vi "Append VI List of SubVIs to Report (string).vi"(0 "report in":refnum<class "NI_report.lvclass">, 2 "image format (jpeg)":enum32{"PNG", "JPEG", "GIF"}(ring)=enum."JPEG", 5 "VI":string, 7 "alignment (default)":T2, 9 "include Express VI configuration information (F)":bool, 11 "error in (no error)":errorcluster, 12 "MS Office parameters":T1) -> (4 "report out":refnum<class "NI_report.lvclass">, 6 "VI name out":string, 8 "start out (Word)":i32, 10 "end out (Word)":i32, 15 "error out":errorcluster)   [LabVIEW 2017, in "NI_ReportGenerationCore.lvlib"]
doc: "Appends a list of subVIs of the VI you specify in <B>VI</B> to a report. The list includes subVI icons, names, and paths. Wire data to the <B>VI</B> input to determine the polymorphic instance to use or manually select the instance."
uses:
  <vilib>/Utility/NIReport.llb/NI_ReportGenerationCore.lvlib
  <vilib>/Utility/NIReport.llb/NI_report.lvclass
  <vilib>/Utility/NIReport.llb/HTML Report Image Alignment.ctl
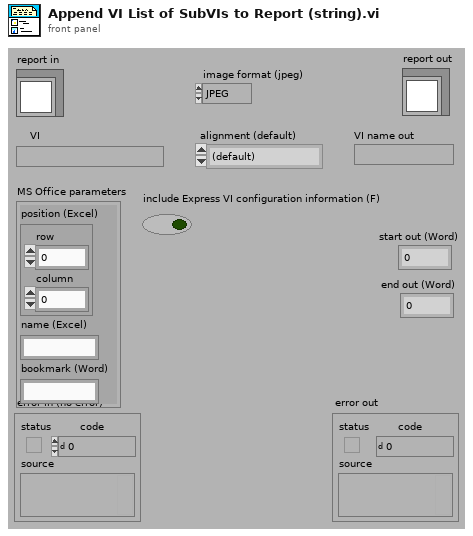
[diagram p1: front panel]
types:
  T1 = cluster{"position (Excel)":cluster{"row":i32, "column":i32}, "name (Excel)":string, "bookmark (Word)":string}
  T2 = typedef "NI_ReportGenerationCore.lvlib/HTML Report Image Alignment.ctl" = enum16{"(default)", "LEFT", "RIGHT", "TOP", "TEXTTOP", "MIDDLE", "ABSMIDDLE", "BASELINE", "BOTTOM", "ABSBOTTOM"}
  T3 = enum32{"invalid app kind", "Development System", "Run Time System", "Student Edition", "Embedded LabVIEW", "Evaluation", "Custom"}
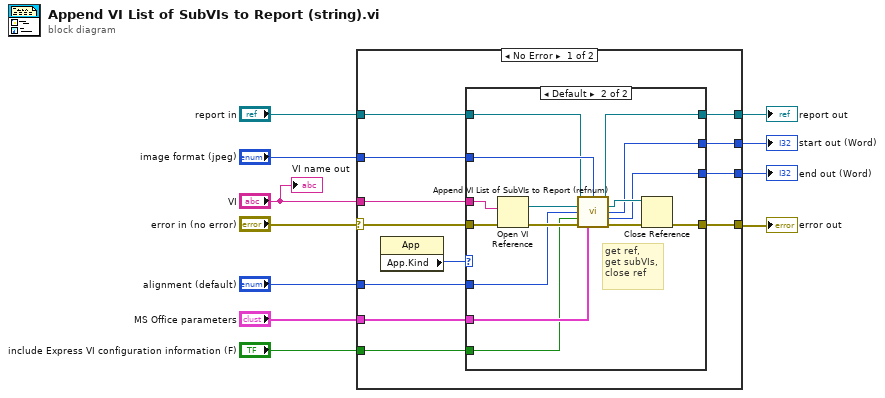
[diagram p0: block diagram]
diagram:
  n1 = case shown="No Error" "error in (no error)" {
    selector: "error in (no error)" -> [w22 w42]
    tunnel: [w17 w42] -> w10
    tunnel: [w21 w41] -> w8
    tunnel: "report in" -> [w15 w41]
    tunnel: "VI" -> [w23 _]
    tunnel: "image format (jpeg)" -> [w18 _]
    tunnel: "alignment (default)" -> [w20 _]
    tunnel: "MS Office parameters" -> [w19 _]
    tunnel: [w13 _] -> w3
    tunnel: [w14 _] -> w2
    tunnel: "include Express VI configuration information (F)" -> [w16 _]
    frame No Error {
      n2 = property class="App"() -> ("App.Kind"=w12:T3)  [unwired: 2 in, 2 out]
      n3 = case shown="Default" w12 {
        tunnel: w23 -> [_ w40]
        tunnel: w22 -> [w24 w39]
        tunnel: [w25 w36] -> w21
        tunnel: w20 -> [_ w35]
        tunnel: w19 -> [_ w34]
        tunnel: w18 -> [_ w33]
        tunnel: [w24 w31] -> w17
        tunnel: w16 -> [_ w29]
        tunnel: w15 -> [w25 w28]
        tunnel: [_ w27] -> w14
        tunnel: [_ w26] -> w13
        frame "Run Time System" {
          # "Do not try to append\nif running in an\nexecutable"
        }
        frame Default {
          # "get ref,\nget subVIs,\nclose ref"
          n4 = Open VI Reference(vi path=w40, error in (no error)=w39) -> (vi reference=w38:refnum<vi>, error out=w37:errorcluster)  [unwired: 4 out]
          n5 = call <vilib>:"Append VI List of SubVIs to Report (refnum).vi"("report in"=w28, "image format (jpeg)"=w33, "VI"=w38, "alignment (default)"=w35, "include Express VI configuration information (F)"=w29, "error in (no error)"=w37, "MS Office parameters"=w34) -> ("report out"=w36:refnum<class "NI_report.lvclass">, "VI out"=w30:refnum<vi>, "start out (Word)"=w27:i32, "end out (Word)"=w26:i32, "error out"=w32:errorcluster)  [unwired: 1 in, 3 out]
          n6 = Close Reference(reference=w30, error in (no error)=w32) -> (error out=w31:errorcluster)
        }
      }
    }
    frame Error {
    }
  }
  "error out" <- w10
  "report out" <- w8
  "start out (Word)" <- w2
  "end out (Word)" <- w3
  "VI name out" <- "VI"
